vi "Ton.vi"(5 "Ton":i32=1000, 7 "input":bool, 11 "error in":errorcluster) -> (4 "elapsed time (ms)":i32, 6 "Pulse":bool, 8 "on":i32, 15 "error out":errorcluster)   [LabVIEW 2022 SP3, in "BinarySignalProcessClass.lvclass"]
uses:
  BinarySignalProcessClass.lvclass
  <vilib>/functionblocks/Counter/Pulse Timer/Pulse Timer.vi
  <vilib>/functionblocks/Counter/Timer Off Delay/Timer Off Delay.vi
  <vilib>/functionblocks/FB Core/FB Core.xnode
  BinarySignalProcessClass.lvclass/BinarySignalProcessClass.ctl
  <vilib>/functionblocks/NI_FunctionBlock Libraries.lvlib
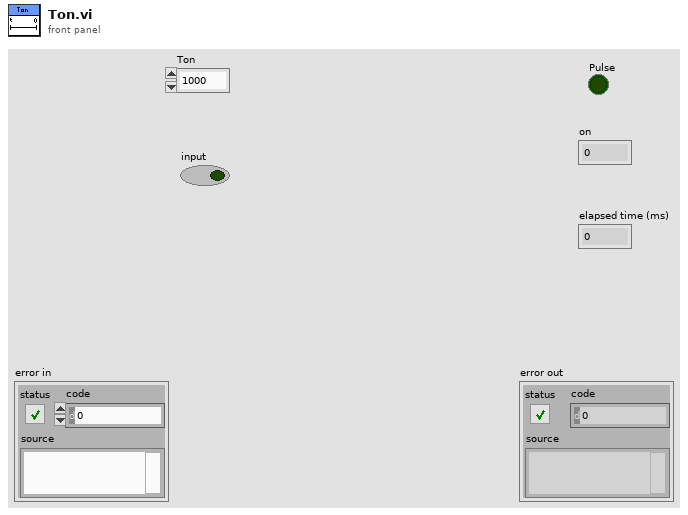
[diagram p1: front panel]
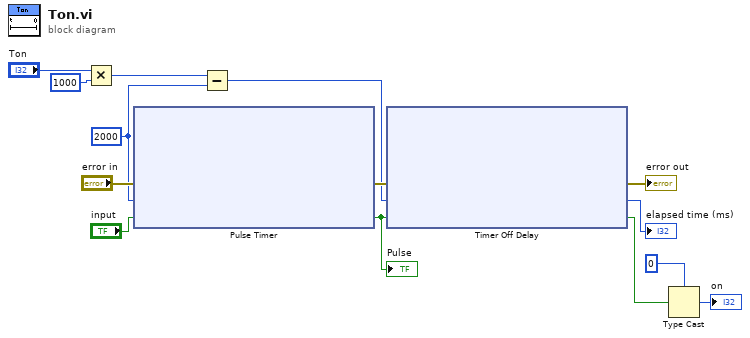
[diagram p0: block diagram]
diagram:
  w2 = 2000 ("preset time (ms)")
  n1 = Multiply(x="Ton", y=1000) -> (x*y=w3:i32)
  n2 = xnode "Pulse Timer"("error in"="error in", "preset time (ms)"=w2, "input"="input") -> ("error out"=w8:errorcluster, "output"=w7:bool)  [unwired: 1 out]
  "Pulse" <- w7
  n3 = Subtract(x=w3, y=w2) -> (x-y=w1:i32)
  n4 = xnode "Timer Off Delay"("error in"=w8, "preset time (ms)"=w1, "input"=w7) -> ("error out"=→"error out":errorcluster, "elapsed time (ms)"=→"elapsed time (ms)":i32, "output"=w5:bool)
  n5 = Type Cast(type=0, x=w5) -> (*(type *) &x=→"on":i32)
